vi "Get Audio File Tags (Core).vi"(8 "error in (no error)":errorcluster, 9 "Read Pictures?":bool, 10 "Encoding":T5, 11 "Path In":string) -> (0 "error out":errorcluster, 1 "Pictures":T1[](array[typedef]), 2 "Tags":T4[](array[typedef]), 3 "Path Out":string)   [LabVIEW 2020, in "G-Audio.lvlib"]
doc: "Retrieve audio file information. Some codecs (mp3) require the entire file be parsed to accurately determine the length, which can take time for very large files.\n\nSupported codecs: flac, mp3, ogg (vorbis), and wav."
uses:
  G-Audio.lvlib
  Controls/Text Encoding.ctl
  Controls/Audio File Tag.ctl
  Controls/Audio File Image.ctl
  Controls/Audio File Image Type.ctl
  <vilib>/picture/picture.llb/imagedata.ctl
  <vilib>/Utility/error.llb/Error Cluster From Error Code.vi
  lib/g_audio_32.dll
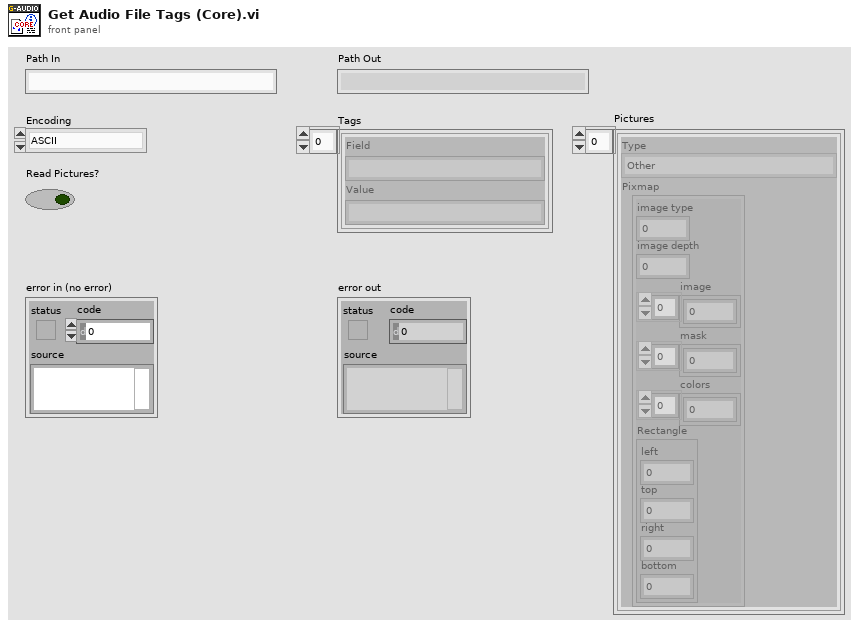
[diagram p1: front panel]
types:
  T1 = typedef "G-Audio.lvlib/Audio File Image.ctl" = cluster{"Type":T2, "Pixmap":T3}
  T2 = typedef "G-Audio.lvlib/Audio File Image Type.ctl" = enum32{"Other", "32x32 pixels 'file icon' (PNG only)", "Other file icon", "Cover (front)", "Cover (back)", "Leaflet page", "Media (e.g. label side of CD)", "Lead artist/lead performer/soloist", "Artist/performer", "Conductor", "Band/Orchestra", "Composer", "Lyricist/text writer", "Recording Location", "During recording", "During performance", "Movie/video screen capture", "A bright coloured fish", "Illustration", "Band/artist logotype", "Publisher/Studio logotype"}
  T3 = typedef "imagedata.ctl" = cluster{"image type":i32, "image depth":i32, "image":u8[], "mask":u8[], "colors":u32[], "Rectangle":cluster{"left":i16, "top":i16, "right":i16, "bottom":i16}}
  T4 = typedef "G-Audio.lvlib/Audio File Tag.ctl" = cluster{"Field":string, "Value":string}
  T5 = typedef "G-Audio.lvlib/Text Encoding.ctl" = enum16{"ASCII", "UTF-8", "UTF-16 LE"}
  T6 = cluster{"uint8_t* data":i32, "uint32_t data_size":u32, "uint32_t type":u32, "uint32_t width":u32, "uint32_t height":u32, "uint32_t depth":u32}
  T7 = cluster{"uint8_t* data":i64, "uint32_t data_size":u32, "uint32_t type":u32, "uint32_t width":u32, "uint32_t height":u32, "uint32_t depth":u32}
  T8 = cluster{"char* field":i32, "char* value":i32, "int32_t field_length":i32, "int32_t value_length":i32}
  T9 = cluster{"char* field":i64, "char* value":i64, "int32_t field_length":i32, "int32_t value_length":i32}
  T10 = cluster{"char* field":i32, "char* value":i32, "int32_t field_length":i32, "int32_t value_length":i32}[]
  T11 = cluster{"uint8_t* data":i32, "uint32_t data_size":u32, "uint32_t type":u32, "uint32_t width":u32, "uint32_t height":u32, "uint32_t depth":u32}[]
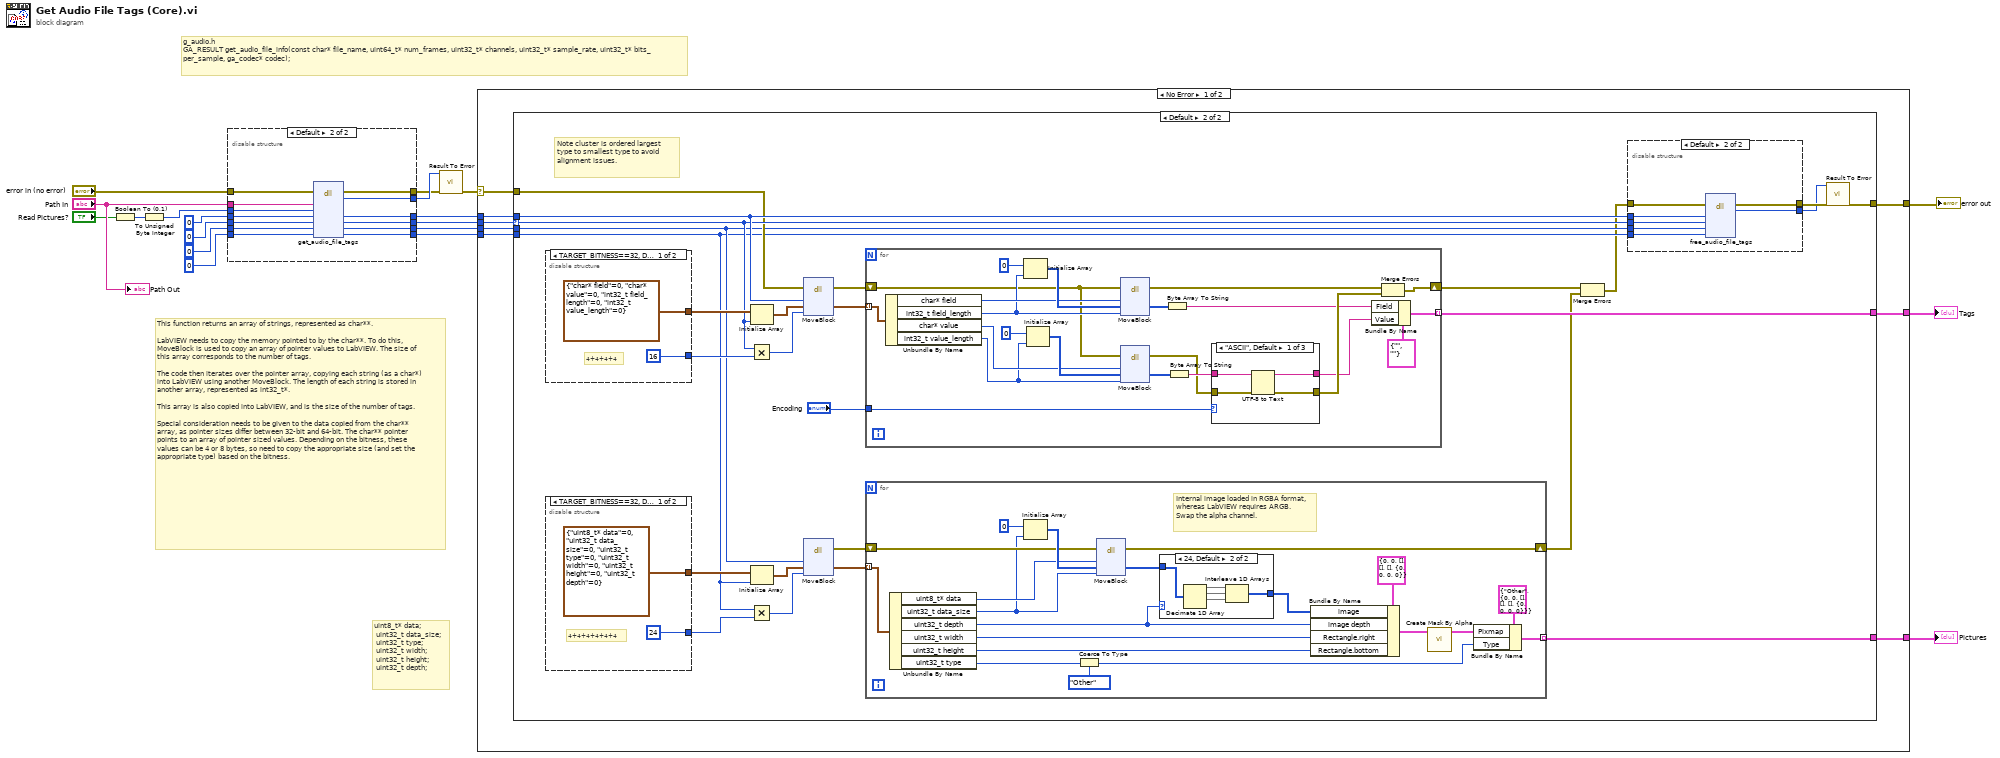
[diagram p0: block diagram]
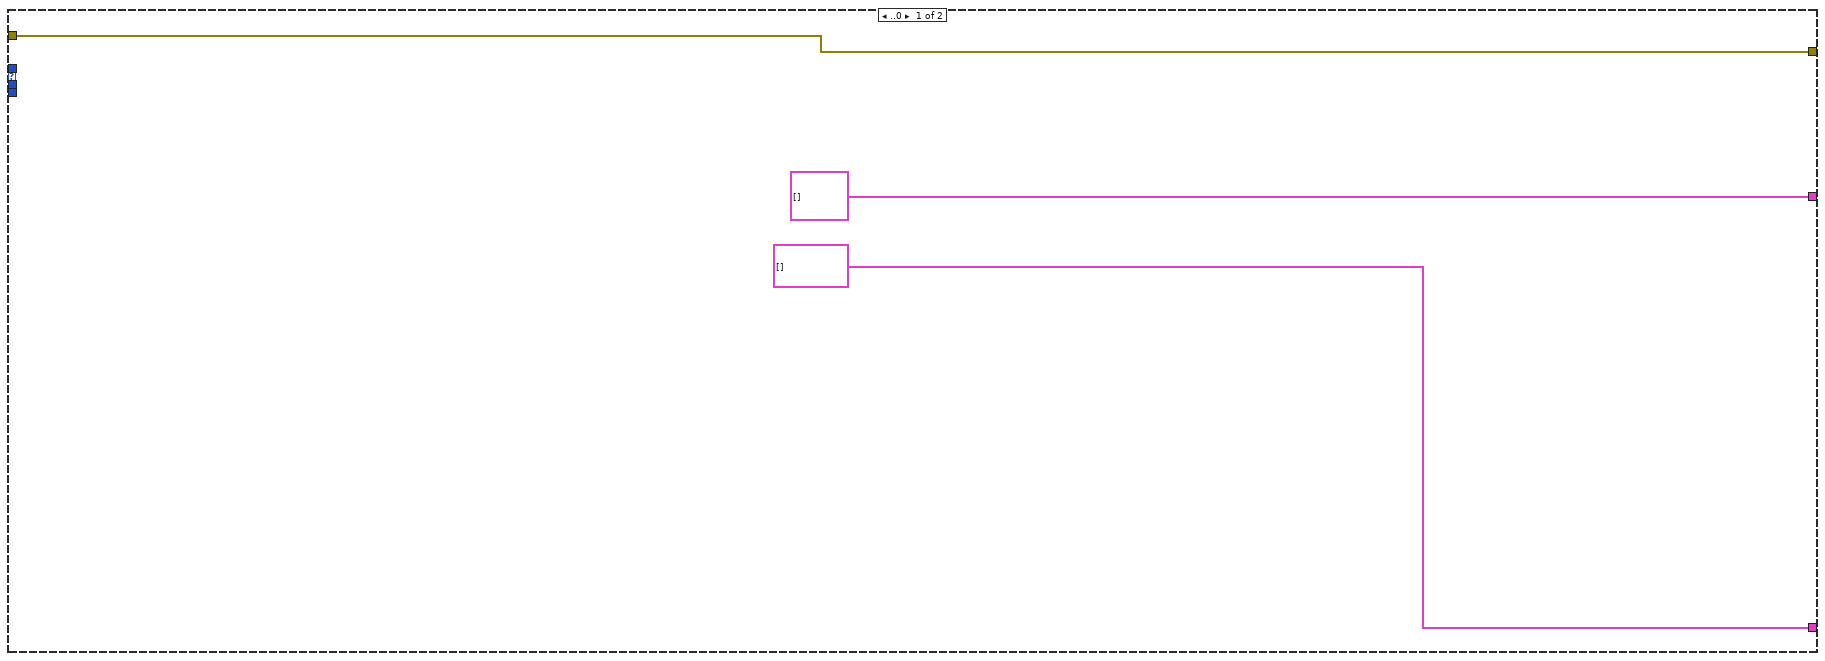
[diagram p2: hidden frame]
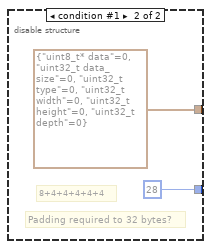
[diagram p3: hidden frame]
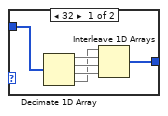
[diagram p4: hidden frame]
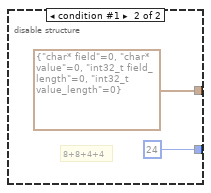
[diagram p5: hidden frame]
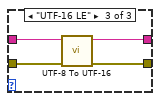
[diagram p7: hidden frame]
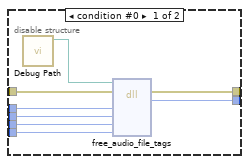
[diagram p8: hidden frame]
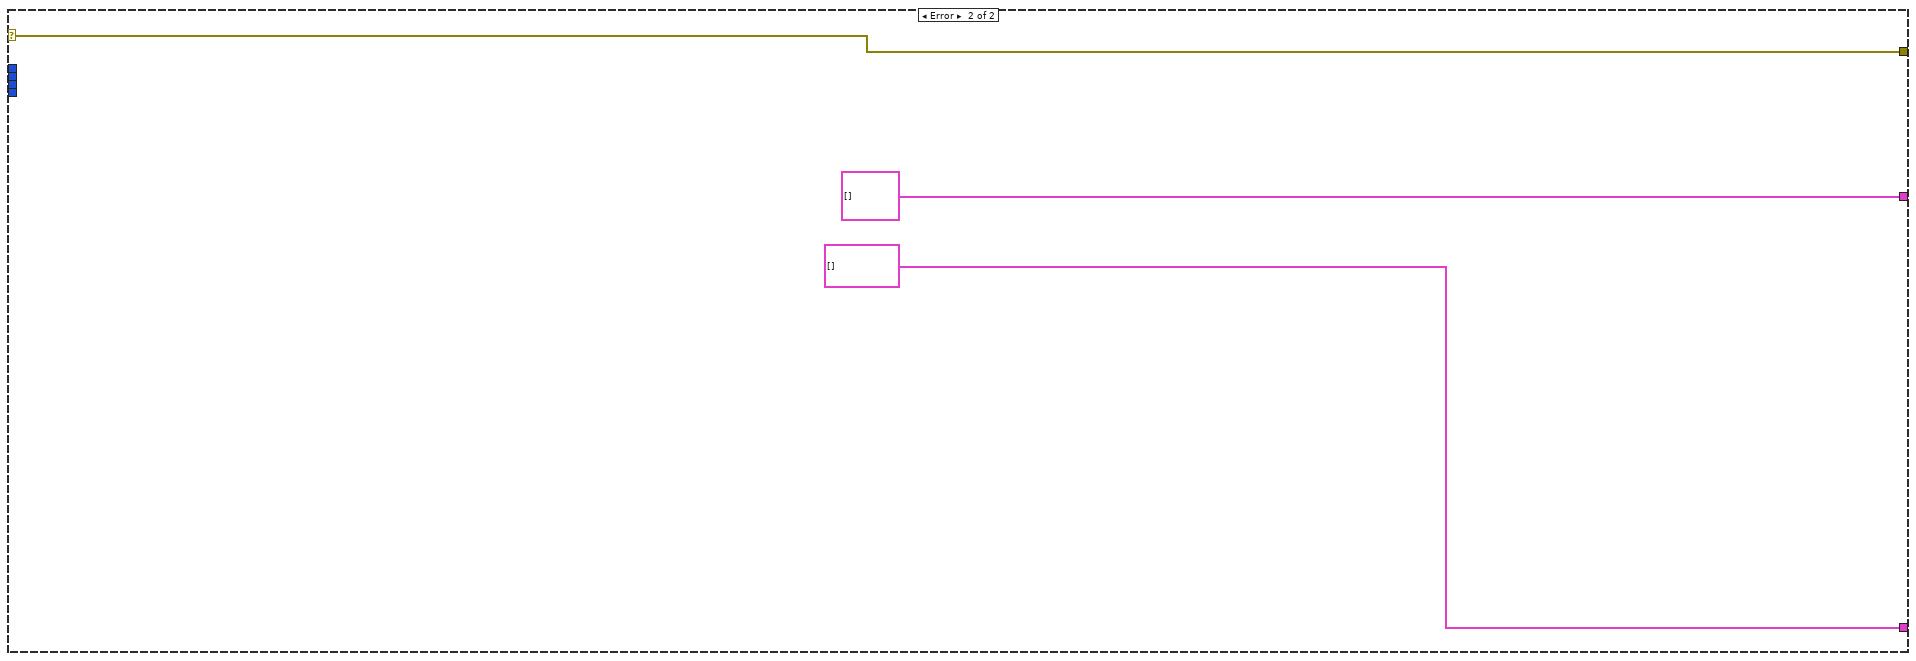
[diagram p9: hidden frame]
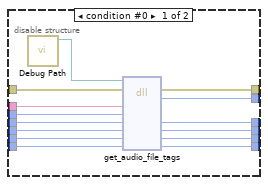
[diagram p10: hidden frame]
diagram:
  # "uint8_t* data;\n\tuint32_t data_size;\n\tuint32_t type;\n\tuint32_t width;\n\tuint32_t height;\n\tuint32_t depth;"
  # "This function returns an array of strings, represented as char**.\n\nLabVIEW needs to copy the memory pointed to by the char**. To do this, MoveBlock is used to copy an array of pointer values to LabVIEW. The size of this array corresponds to the number of tags.\n\nThe code then iterates over the pointer array, copying each string (as a char*) into LabVIEW using another MoveBlock. The length of each string is stored in another array, represented as int32_t*.\n\nThis array is also copied into LabVIEW, and is the size of the number of tags.\n\nSpecial consideration needs to be given to the data copied from the char** array, as pointer sizes differ between 32-bit and 64-bit. The char** pointer points to an array of pointer sized values. Depending on the bitness, these values can be 4 or 8 bytes, so need to copy the appropriate size (and set the appropriate type) based on the bitness."
  # "g_audio.h\nGA_RESULT get_audio_file_info(const char* file_name, uint64_t* num_frames, uint32_t* channels, uint32_t* sample_rate, uint32_t* bits_per_sample, ga_codec* codec);"
  n1 = Boolean To (0,1)(Boolean="Read Pictures?") -> (0, 1=w2:i16)
  n2 = To Unsigned Byte Integer(number=w2) -> (unsigned 8bit integer=w1:u8)
  n3 = disable-structure shown="Default" {
    disable-tunnel: [w28 w46] -> w14
    disable-tunnel: [w27 w45] -> w15
    disable-tunnel: [w32 w44] -> w12
    disable-tunnel: 0 ("tags") -> [w23 w39]
    disable-tunnel: i64 0 ("count") -> [w24 w40]
    disable-tunnel: "error in (no error)" -> [w31 w43]
    disable-tunnel: "Path In" -> [w30 w42]
    disable-tunnel: [w29 w41] -> w13
    disable-tunnel: [w26 w35] -> w6
    disable-tunnel: [w25 w34] -> w5
    disable-tunnel: i64 0 ("count") -> [w22 w37]
    disable-tunnel: 0 ("tags") -> [w21 w36]
    disable-tunnel: w1 -> [w20 w38]
    frame condition #0 {
      n4 = call "Debug Path.vi"() -> ("Debug Path"=w33:path)  [unwired: 11 in]
      n5 = dll-call lib="?" fn="get_audio_file_tags"(path in=w33, error in=w31, "file_name"=w30, "read_pictures"=w20, "tags"=w24, "tag_count"=w23, "pictures"=w22, "picture_count"=w21) -> (error out=w32:errorcluster, "result"=w29:i32, "tags"=w28:i64, "tag_count"=w27:i32, "pictures"=w26:i64, "picture_count"=w25:i32)  [unwired: 3 in, 1 out]
    }
    frame condition #1 (active) {
      n6 = dll-call lib="C:/github/dataflowg/g-audio/src/LabVIEW/G-Audio/lib/g_audio_*.*" fn="get_audio_file_tags"(error in=w43, "file_name"=w42, "read_pictures"=w38, "tags"=w40, "tag_count"=w39, "pictures"=w37, "picture_count"=w36) -> (error out=w44:errorcluster, "result"=w41:i32, "tags"=w46:i64, "tag_count"=w45:i32, "pictures"=w35:i64, "picture_count"=w34:i32)  [unwired: 4 in, 1 out]
    }
  }
  n7 = call "Result To Error.vi"("error in (no error)"=w12, "Result Code"=w13) -> ("error out"=w11:errorcluster)  [unwired: 9 in]
  n8 = case shown="No Error" w11 {
    selector: w11 -> [w51 w172]
    tunnel: [w54 w172] -> w19
    tunnel: [w53 T4[] []] -> w9
    tunnel: w15 -> [w50 _]
    tunnel: w14 -> [w52 _]
    tunnel: w6 -> [w49 _]
    tunnel: w5 -> [w48 _]
    tunnel: [w47 T1[] []] -> w4
    frame No Error {
      n9 = case shown="Default" w50 {
        selector: w50 -> [_ w75]
        tunnel: [w57 w71] -> w54
        tunnel: [T4[] [] w70] -> w53
        tunnel: w52 -> [_ w78]
        tunnel: w51 -> [w57 w73]
        tunnel: w49 -> [_ w62]
        tunnel: w48 -> [_ w61]
        tunnel: [T1[] [] w63] -> w47
        frame ..0 {
        }
        frame Default {
          # "Note cluster is ordered largest type to smallest type to avoid alignment issues."
          n10 = disable-structure shown="TARGET_BITNESS==32, Default" {
            disable-tunnel: [T8 {"char* field"=0, "char* value"=0, "int32_t field_length"=0, "int32_t value_length"=0} T9 {"char* field"=0, "char* value"=0, "int32_t field_length"=0, "int32_t value_length"=0}] -> w83
            disable-tunnel: [16 ("x") 24 ("x")] -> w79
            frame condition #0 (active) {
              # "4+4+4+4"
            }
            frame condition #1 {
              # "8+8+4+4"
            }
          }
          n11 = disable-structure shown="TARGET_BITNESS==32, Default" {
            disable-tunnel: [T6 {"uint8_t* data"=0, "uint32_t data_size"=0, "uint32_t type"=0, "uint32_t width"=0, "uint32_t height"=0, "uint32_t depth"=0} T7 {"uint8_t* data"=0, "uint32_t data_size"=0, "uint32_t type"=0, "uint32_t width"=0, "uint32_t height"=0, "uint32_t depth"=0}] -> w64
            disable-tunnel: [24 ("x") 28 ("x")] -> w68
            frame condition #0 (active) {
              # "4+4+4+4+4+4"
            }
            frame condition #1 {
              # "Padding required to 32 bytes?"
              # "8+4+4+4+4+4"
            }
          }
          n12 = Initialize Array(w83, w75) -> (w82:T10)
          n13 = Multiply(x=w75, y=w79) -> (x*y=w81:i32)
          n14 = Initialize Array(w64, w61) -> (w65:T11)
          n15 = Multiply(x=w61, y=w68) -> (x*y=w66:i32)
          n16 = dll-call lib="LabVIEW" fn="MoveBlock"(error in=w73, "Address (Pointer)"=w78, "Destination"=w82, "Size"=w81) -> (error out=w72:errorcluster, "Destination"=w80:T10)  [unwired: 5 in, 1 out]
          n17 = dll-call lib="LabVIEW" fn="MoveBlock"("Address (Pointer)"=w62, "Destination"=w65, "Size"=w66) -> (error out=w69:errorcluster, "Destination"=w67:T11)  [unwired: 6 in, 1 out]
          n18 = for {
            tunnel: w80 -> [w141] mode=indexing
            tunnel: [w124] -> w70 mode=indexing
            tunnel: "Encoding" -> [w132]
            shift-right: [w127] -> w60
            shift-left: w72 -> [w131]
            n19 = Unbundle By Name(w141) -> ("char* field"=w140:i32, "int32_t field_length"=w139:i32, "char* value"=w135:i32, "int32_t value_length"=w134:i32)
            n20 = Initialize Array(u8 0 ("element"), w139) -> (w143:u8[])
            n21 = Initialize Array(u8 0 ("element"), w134) -> (w137:u8[])
            n22 = dll-call lib="LabVIEW" fn="MoveBlock"(error in=w131, "Address (Pointer)"=w140, "Destination"=w143, "Size"=w139) -> (error out=w130:errorcluster, "Destination"=w142:u8[])  [unwired: 5 in, 1 out]
            n23 = dll-call lib="LabVIEW" fn="MoveBlock"(error in=w131, "Address (Pointer)"=w135, "Destination"=w137, "Size"=w134) -> (error out=w129:errorcluster, "Destination"=w138:u8[])  [unwired: 5 in, 1 out]
            n24 = Byte Array To String(unsigned byte array=w142) -> (string=w126:string)
            n25 = Byte Array To String(unsigned byte array=w138) -> (string=w133:string)
            n26 = case shown="\"ASCII\", Default" w132 {
              tunnel: w133 -> [w148 w150 w154]
              tunnel: [w147 w150 w153] -> w125
              tunnel: w129 -> [w146 w149 w152]
              tunnel: [w145 w149 w151] -> w128
              frame "ASCII", Default {
                n27 = UTF-8 to Text(8:w146, 11:w148) -> (0:w145:errorcluster, 3:w147:string)  [unwired: 1 in]
              }
              frame "UTF-8" {
                # "Tags are returned in UTF-8 format."
              }
              frame "UTF-16 LE" {
                n28 = call "UTF-8 To UTF-16.vi"("error in (no error)"=w152, "UTF-8"=w154) -> ("error out"=w151:errorcluster, "UTF-16"=w153:string)  [unwired: 8 in]
              }
            }
            n29 = Bundle By Name(cluster=T4 {"Field"="", "Value"=""} ("Tag"), "Field"=w126, "Value"=w125) -> (w124:T4)
            n30 = Merge Errors(w130, w128) -> (w127:errorcluster)
          }
          n31 = for {
            tunnel: w67 -> [w105] mode=indexing
            shift-right: [w102] -> w59
            shift-left: w69 -> [w103]
            tunnel: [w89] -> w63 mode=indexing
            # "Internal image loaded in RGBA format, whereas LabVIEW requires ARGB. Swap the alpha channel."
            n32 = Unbundle By Name(w105) -> ("uint8_t* data"=w104:i32, "uint32_t data_size"=w97:u32, "uint32_t depth"=w88:u32, "uint32_t width"=w101:u32, "uint32_t height"=w100:u32, "uint32_t type"=w99:u32)
            n33 = Initialize Array(u8 0 ("element"), w97) -> (w106:u8[])
            n34 = Coerce To Type(0:w99, 1:Audio_File_Image_Type."Other" ("Type")) -> (2:w90:T2)
            n35 = dll-call lib="LabVIEW" fn="MoveBlock"(error in=w103, "Address (Pointer)"=w104, "Destination"=w106, "Size"=w97) -> (error out=w102:errorcluster, "Destination"=w96:u8[])  [unwired: 5 in, 1 out]
            n36 = case shown="24, Default" w88 {
              tunnel: w96 -> [w113 w118]
              tunnel: [w112 w117] -> w95
              frame 32 {
                n37 = Decimate 1D Array(w113) -> (w111:u8[], w110:u8[], w109:u8[], w108:u8[])
                n38 = Interleave 1D Arrays(w108, w111, w110, w109) -> (w112:u8[])
              }
              frame 24, Default {
                n39 = Decimate 1D Array(w118) -> (w116:u8[], w115:u8[], w114:u8[])  [unwired: 1 out]
                n40 = Interleave 1D Arrays(w116, w115, w114) -> (w117:u8[])
              }
            }
            n41 = Bundle By Name(cluster=T3 {"image type"=0, "image depth"=0, "image"=[], "mask"=[], "colors"=[], "Rectangle"={"left"=0, "top"=0, "right"=0, "bottom"=0}} ("Pixmap"), "image"=w95, "image depth"=w88, "Rectangle.right"=w101, "Rectangle.bottom"=w100) -> (w93:T3)
            n42 = call <vilib>:"Create Mask By Alpha.vi"("image data"=w93) -> ("masked image data"=w91:T3)  [unwired: 10 in]
            n43 = Bundle By Name(cluster=T1 {"Type"=enum."Other", "Pixmap"={"image type"=0, "image depth"=0, "image"=[], "mask"=[], "colors"=[], "Rectangle"={"left"=0, "top"=0, "right"=0, "bottom"=0}}} ("Image Tag"), "Pixmap"=w91, "Type"=w90) -> (w89:T1)
          }
          n44 = Merge Errors(w60, w59) -> (w58:errorcluster)
          n45 = disable-structure shown="Default" {
            disable-tunnel: w75 -> [w161 w169]
            disable-tunnel: w58 -> [w160 w168]
            disable-tunnel: w78 -> [w159 w167]
            disable-tunnel: [w158 w166] -> w77
            disable-tunnel: [w157 w165] -> w76
            disable-tunnel: w62 -> [w156 w164]
            disable-tunnel: w61 -> [w155 w163]
            frame condition #0 {
              n46 = call "Debug Path.vi"() -> ("Debug Path"=w162:path)  [unwired: 11 in]
              n47 = dll-call lib="?" fn="free_audio_file_tags"(path in=w162, error in=w160, "tags"=w159, "tag_count"=w161, "pictures"=w156, "picture_count"=w155) -> (error out=w158:errorcluster, "result"=w157:i32)  [unwired: 5 in, 1 out]
            }
            frame condition #1 (active) {
              n48 = dll-call lib="C:/github/dataflowg/g-audio/src/LabVIEW/G-Audio/lib/g_audio_*.*" fn="free_audio_file_tags"(error in=w168, "tags"=w167, "tag_count"=w169, "pictures"=w164, "picture_count"=w163) -> (error out=w166:errorcluster, "result"=w165:i32)  [unwired: 6 in, 1 out]
            }
          }
          n49 = call "Result To Error.vi"("error in (no error)"=w77, "Result Code"=w76) -> ("error out"=w71:errorcluster)  [unwired: 9 in]
        }
      }
    }
    frame Error {
    }
  }
  "error out" <- w19
  "Tags" <- w9
  "Pictures" <- w4
  "Path Out" <- "Path In"
